vi "GCode File to Array.vi"(11 "File Path":path) -> (3 "G-Code Array":string[](array[string]))   [LabVIEW 2017]
doc: "Converts a G-Code file into a one dimensional array where each row is a G-Code command. \n\n<B>Inputs</B>: \n- File Path: G-Code file to be converted into array. \n\n<B>Outputs</B>: \n- G-Code Array: One dimensional array. Each row is a G-Code command."
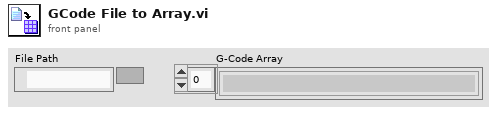
[diagram p1: front panel]
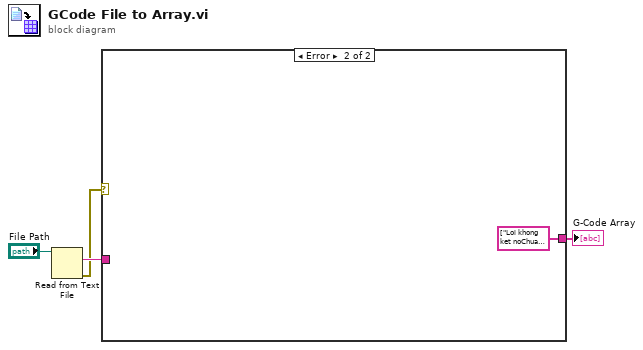
[diagram p0: block diagram]
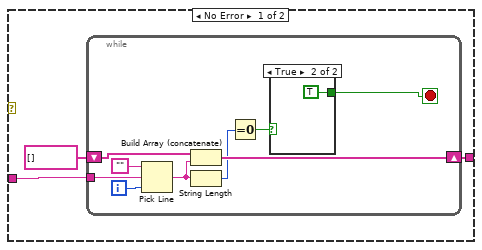
[diagram p2: hidden frame]
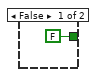
[diagram p3: hidden frame]
diagram:
  n1 = Read from Text File(file (use dialog)="File Path") -> (text=w3:string, error out=w1:errorcluster)  [unwired: 3 in, 2 out]
  n2 = case shown="Error" w1 {
    tunnel: w3 -> [w7 _]
    tunnel: [w6 string[] ["Loi khong ket noChua Chon File"]] -> w2
    frame No Error {
      n3 = while {
        shift-right: [w14] -> w6
        shift-left: string[] [] -> [w15]
        tunnel: w7 -> [w9]
        i -> [w16]
        stop <- w8 stop-if-true
        n4 = Pick Line(string ("")="", multi-line string=w9, line index=w16) -> (output string=w12:string)
        n5 = Build Array (concatenate)(w15, w12) -> (w14:string[])
        n6 = String Length(string=w12) -> (length=w11:i32)
        n7 = Equal To 0?(x=w11) -> (x = 0?=w10:bool)
        n8 = case shown="True" w10 {
          tunnel: [FALSE TRUE] -> w8
          frame False {
          }
          frame True {
          }
        }
      }
    }
    frame Error {
    }
  }
  "G-Code Array" <- w2
